vi "MGI Coerce Rect into Bounds.vi"(2 "Bounds":T1, 3 "Rect":T2) -> (0 "Rect Resized?":bool, 1 "Coerced Rect":T2)   [LabVIEW 2020]
doc: "Coerce the specified rect to fit within the bounds supplied. If the rect is larger than the bounds it will be resized to fit.\n\nAuthored by Stephen Moore\nsupport@mooregoodideas.com\nwww.mooregoodideas.com\n\nCopyright (c) 2010, Moore Good Ideas, Inc.\n\nAll rights reserved.\n\nRedistribution and use in source and binary forms, with or without modification, are permitted provided that the following conditions are met:\n\n * Redistributions of source code must retain the above copyright notice, this list of conditions and the following disclaimer.\n * Redistributions in binary form must reproduce the above copyright notice, this list of conditions and the following disclaimer in the documentation and/or other materials provided with the distribution.\n * Neither the name of Moore Good Ideas, Inc. nor the names of its contributors may be used to endorse or promote products derived from this software without specific prior written permission.\n\nTHIS SOFTWARE IS PROVIDED BY THE COPYRIGHT HOLDERS AND CONTRIBUTORS \"AS IS\" AND ANY EXPRESS OR IMPLIED WARRANTIES, INCLUDING, BUT NOT LIMITED TO, THE IMPLIED WARRANTIES OF MERCHANTABILITY AND FITNESS FOR A PARTICULAR PURPOSE ARE DISCLAIMED. IN NO EVENT SHALL THE COPYRIGHT OWNER OR CONTRIBUTORS BE LIABLE FOR ANY DIRECT, INDIRECT, INCIDENTAL, SPECIAL, EXEMPLARY, OR CONSEQUENTIAL DAMAGES (INCLUDING, BUT NOT LIMITED TO, PROCUREMENT OF SUBSTITUTE GOODS OR SERVICES; LOSS OF USE, DATA, OR PROFITS; OR BUSINESS INTERRUPTION) HOWEVER CAUSED AND ON ANY THEORY OF LIABILITY, WHETHER IN CONTRACT, STRICT LIABILITY, OR TORT (INCLUDING NEGLIGENCE OR OTHERWISE) ARISING IN ANY WAY OUT OF THE USE OF THIS SOFTWARE, EVEN IF ADVISED OF THE POSSIBILITY OF SUCH DAMAGE."
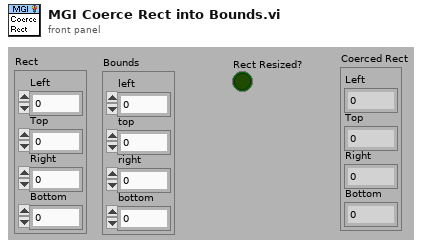
[diagram p1: front panel]
types:
  T1 = cluster{"left":i16, "top":i16, "right":i16, "bottom":i16}
  T2 = cluster{"Left":i16, "Top":i16, "Right":i16, "Bottom":i16}
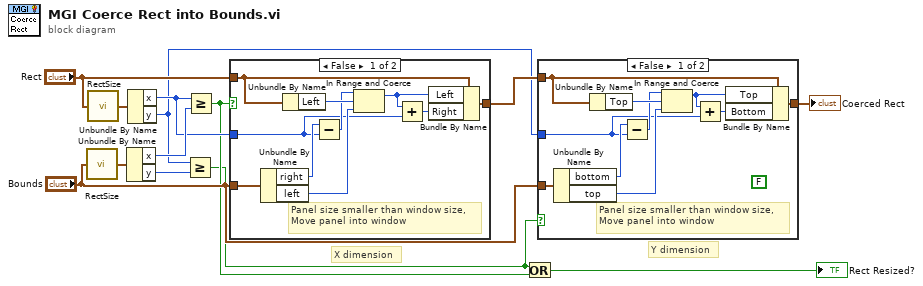
[diagram p0: block diagram]
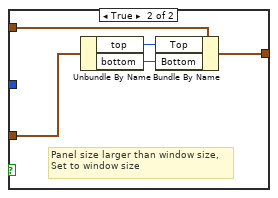
[diagram p2: hidden frame]
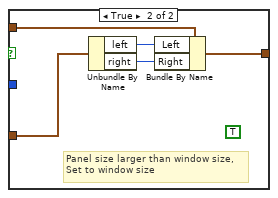
[diagram p3: hidden frame]
diagram:
  # "X dimension"
  # "Y dimension"
  n1 = call <vilib>:"RectSize.vi"("rect"="Bounds") -> ("point"=w11:cluster{"x":i16, "y":i16})
  n2 = call <vilib>:"RectSize.vi"("rect"="Rect") -> ("point"=w12:cluster{"x":i16, "y":i16})
  n3 = Unbundle By Name(w11) -> ("x"=w10:i16, "y"=w7:i16)
  n4 = Unbundle By Name(w12) -> ("x"=w9:i16, "y"=w6:i16)
  n5 = Greater Or Equal?(x=w6, y=w7) -> (x >= y?=w1:bool)
  n6 = Greater Or Equal?(x=w9, y=w10) -> (x >= y?=w3:bool)
  n7 = case shown="False" w3 {
    tunnel: "Bounds" -> [w23 w24]
    tunnel: "Rect" -> [w15 w25]
    tunnel: w9 -> [w16 _]
    tunnel: [w14 w26] -> w8
    frame False {
      # "Panel size smaller than window size,\nMove panel into window"
      n8 = Unbundle By Name(w23) -> ("right"=w19:i16, "left"=w21:i16)
      n9 = Unbundle By Name(w15) -> ("Left"=w22:i16)
      n10 = Subtract(x=w19, y=w16) -> (x-y=w20:i16)
      n11 = In Range and Coerce(upper limit=w20, x=w22, lower limit=w21) -> (coerced(x)=w18:i16)  [unwired: 1 out]
      n12 = Add(x=w18, y=w16) -> (x+y=w17:i16)
      n13 = Bundle By Name(cluster=w15, "Left"=w18, "Right"=w17) -> (w14:T2)
    }
    frame True {
      (unwired) TRUE
      # "Panel size larger than window size,\nSet to window size"
      n14 = Unbundle By Name(w24) -> ("left"=w28:i16, "right"=w27:i16)
      n15 = Bundle By Name(cluster=w25, "Left"=w28, "Right"=w27) -> (w26:T2)
    }
  }
  n16 = Or(x=w1, y=w3) -> (x .or. y?=→"Rect Resized?":bool)
  n17 = case shown="False" w1 {
    tunnel: "Bounds" -> [w38 w43]
    tunnel: w8 -> [w30 w39]
    tunnel: w6 -> [w31 _]
    tunnel: [w29 w40] -> w4
    frame False {
      (unwired) FALSE
      # "Panel size smaller than window size,\nMove panel into window"
      n18 = Unbundle By Name(w38) -> ("bottom"=w34:i16, "top"=w36:i16)
      n19 = Unbundle By Name(w30) -> ("Top"=w37:i16)
      n20 = Subtract(x=w34, y=w31) -> (x-y=w35:i16)
      n21 = In Range and Coerce(upper limit=w35, x=w37, lower limit=w36) -> (coerced(x)=w33:i16)  [unwired: 1 out]
      n22 = Add(x=w33, y=w31) -> (x+y=w32:i16)
      n23 = Bundle By Name(cluster=w30, "Top"=w33, "Bottom"=w32) -> (w29:T2)
    }
    frame True {
      # "Panel size larger than window size,\nSet to window size"
      n24 = Unbundle By Name(w43) -> ("top"=w42:i16, "bottom"=w41:i16)
      n25 = Bundle By Name(cluster=w39, "Top"=w42, "Bottom"=w41) -> (w40:T2)
    }
  }
  "Coerced Rect" <- w4
